vi "Resize_Image.vi"(0 "Draw_Area":T2, 5 "Image_Property":T1) -> (4 "Numeric":sgl)   [LabVIEW 2023]
doc: "This VI Resize the Image"
uses:
  <vilib>/Utility/miscctls.llb/LVBoundsTypeDef.ctl
  <vilib>/picture/picture.llb/imagedata.ctl
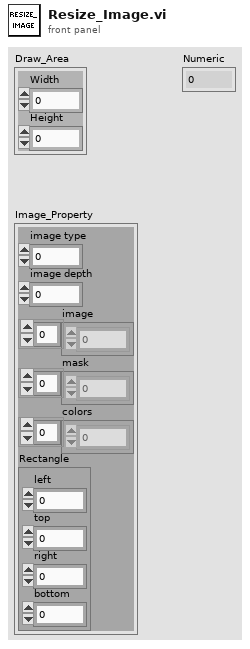
[diagram p1: front panel]
types:
  T1 = typedef "imagedata.ctl" = cluster{"image type":i32, "image depth":i32, "image":u8[], "mask":u8[], "colors":u32[], "Rectangle":cluster{"left":i16, "top":i16, "right":i16, "bottom":i16}}
  T2 = typedef "LVBoundsTypeDef.ctl" = cluster{"Width":u32, "Height":u32}
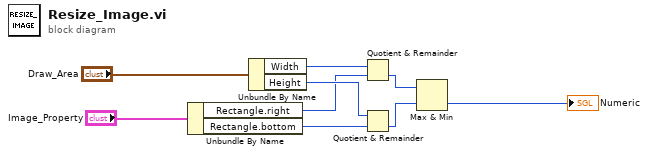
[diagram p0: block diagram]
diagram:
  n1 = Unbundle By Name("Image_Property") -> ("Rectangle.right"=w3:i16, "Rectangle.bottom"=w2:i16)
  n2 = Unbundle By Name("Draw_Area") -> ("Width"=w7:u32, "Height"=w6:u32)
  n3 = Quotient & Remainder(x=w7, y=w3) -> (floor(x/y)=w4:u32)  [unwired: 1 out]
  n4 = Quotient & Remainder(x=w6, y=w2) -> (floor(x/y)=w5:u32)  [unwired: 1 out]
  n5 = Max & Min(x=w4, y=w5) -> (min(x,y)=→"Numeric":u32)  [unwired: 1 out]
